vi "AirFow Characteistics.vi"(0 "Numeric in":dbl, 1 "Viscosity (Pa-s)":dbl, 2 "Density (kg/m^3) 2":dbl, 3 "Velocity (m/s) 2":dbl, 4 "Viscosity (Pa-s) 2":dbl, 5 "Average 3":dbl, 6 "Velocity (m/s)":dbl, 7 "Average":dbl, 8 "Stack Inner Diameter (m)":dbl, 9 "Average 2":dbl, 10 "Density (kg/m^3)":dbl) -> (11 "Friction Factor 2":dbl, 12 "BC Reynolds":dbl, 13 "Friction Factor":dbl, 14 "AB Reynolds":dbl, 15 "AB f":dbl, 16 "BC f":dbl, 17 "CD Reynolds":dbl, 18 "CD f":dbl, 19 "Numeric out":dbl)   [LabVIEW 2019]
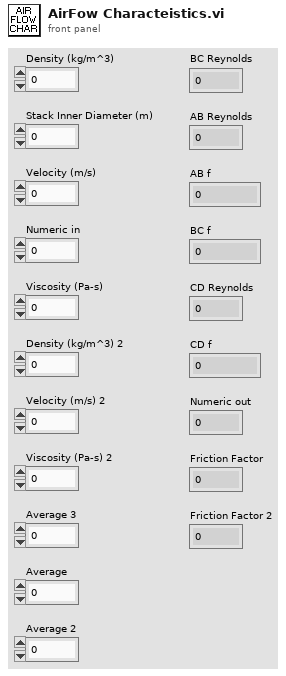
[diagram p1: front panel]
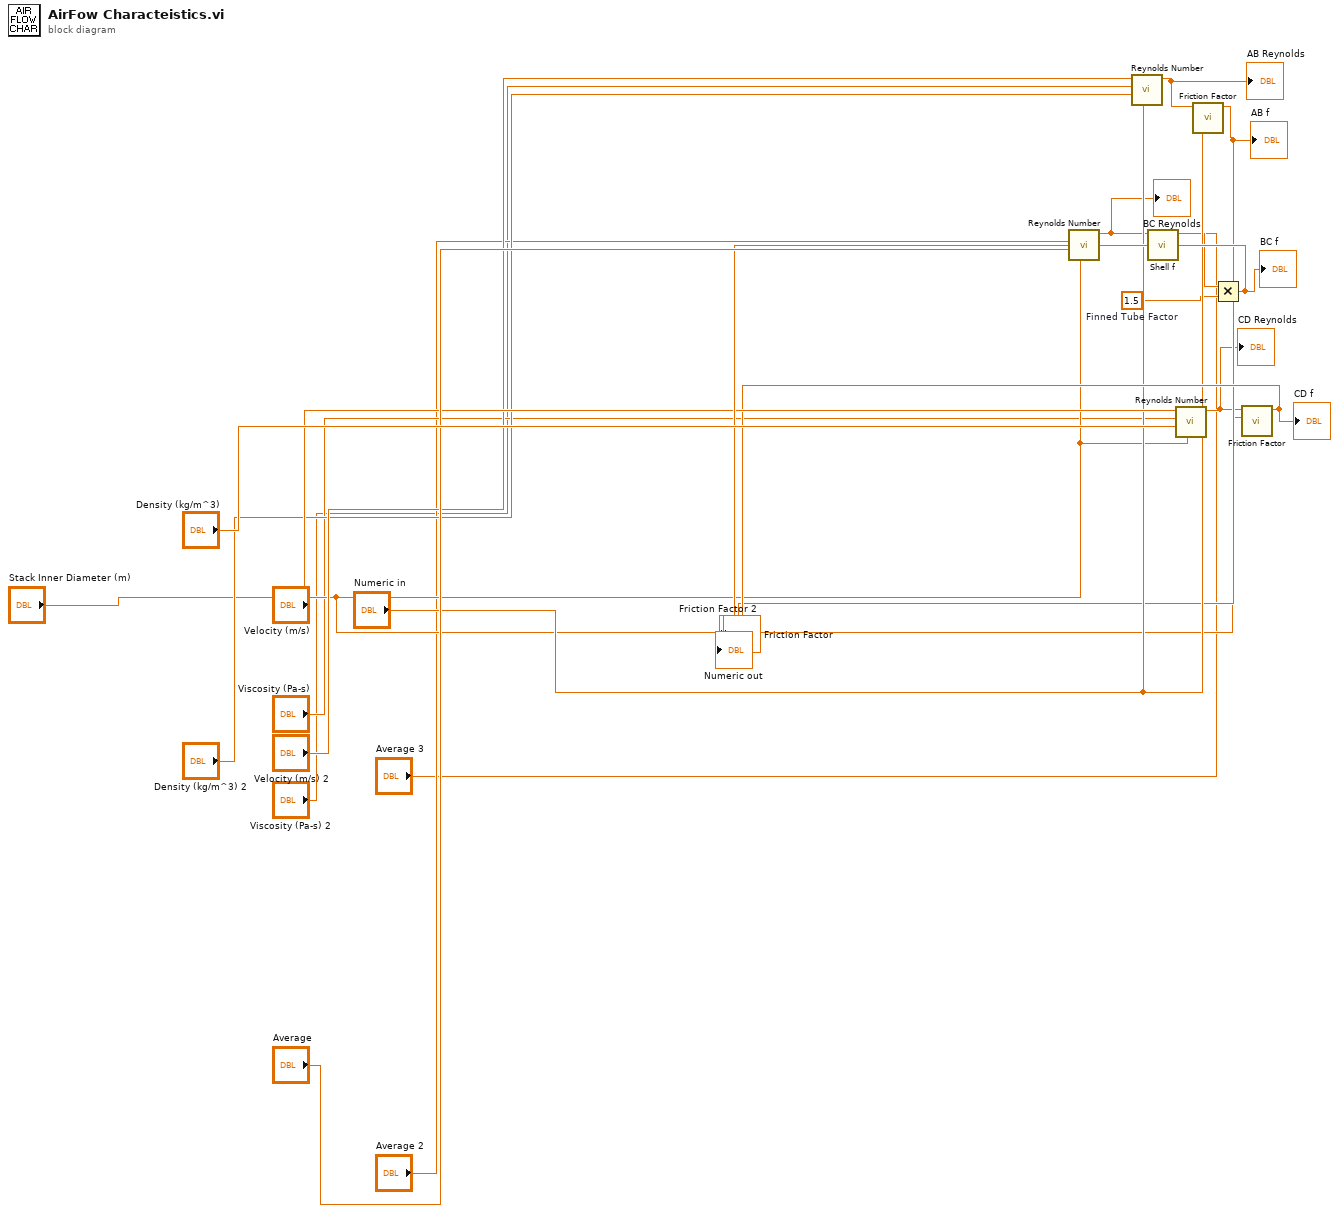
[diagram p0: block diagram]
diagram:
  w9 = 1.5  # Finned Tube Factor
  n1 = call "Reynolds Number.vi"("Effective Length (m)"="Stack Inner Diameter (m)", "Density (kg/m^3)"="Average", "Viscosity (Pa-s)"="Average 2", "Velocity (m/s)"="Average 3") -> ("Reynolds Number"=w5:dbl)  [unwired: 7 in]
  "BC Reynolds" <- w5
  n2 = call "Reynolds Number.vi"("Effective Length (m)"="Numeric in", "Density (kg/m^3)"="Density (kg/m^3) 2", "Viscosity (Pa-s)"="Viscosity (Pa-s) 2", "Velocity (m/s)"="Velocity (m/s) 2") -> ("Reynolds Number"=w1:dbl)  [unwired: 7 in]
  "AB Reynolds" <- w1
  n3 = call "Shell f.vi"("Reynolds Number"=w5) -> ("Numeric"=w10:dbl)  [unwired: 10 in]
  n4 = call "Reynolds Number.vi"("Effective Length (m)"="Stack Inner Diameter (m)", "Density (kg/m^3)"="Density (kg/m^3)", "Viscosity (Pa-s)"="Viscosity (Pa-s)", "Velocity (m/s)"="Velocity (m/s)") -> ("Reynolds Number"=w7:dbl)  [unwired: 7 in]
  "CD Reynolds" <- w7
  n5 = call "Friction Factor.vi"("Effective Length"="Numeric in", "Reynolds Number"=w1) -> ("Friction Factor"=→"AB f" →"Friction Factor 2":dbl)  [unwired: 9 in]
  n6 = Multiply(x=w10, y=w9) -> (x*y=→"BC f" →"Numeric out":dbl)
  n7 = call "Friction Factor.vi"("Effective Length"="Stack Inner Diameter (m)", "Reynolds Number"=w7) -> ("Friction Factor"=→"CD f" →"Friction Factor":dbl)  [unwired: 9 in]
